vi "Close.vi"(8 "error in (no error)":errorcluster, 11 "HOTCOIL Settings":T1) -> (0 "error out":errorcluster, 3 "HOTCOIL Settings":T1)   [LabVIEW 2021, in "HotCoil.lvlib"]
uses:
  HotCoil.lvlib
  HotCoil Settings.ctl
panel:
  out "Array 2":string[](array[string])
  out "Array":string[](array[string])
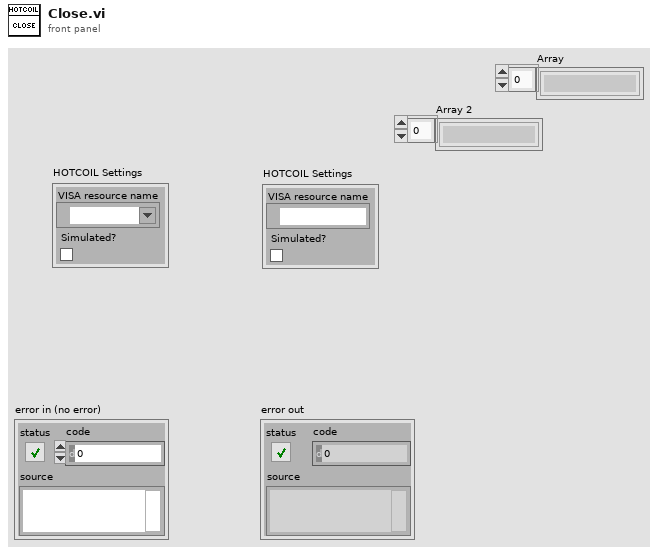
[diagram p1: front panel]
types:
  T1 = typedef "HotCoil.lvlib/HotCoil Settings.ctl" = cluster{"VISA resource name":refnum<visa-resource-name>, "Simulated?":bool}
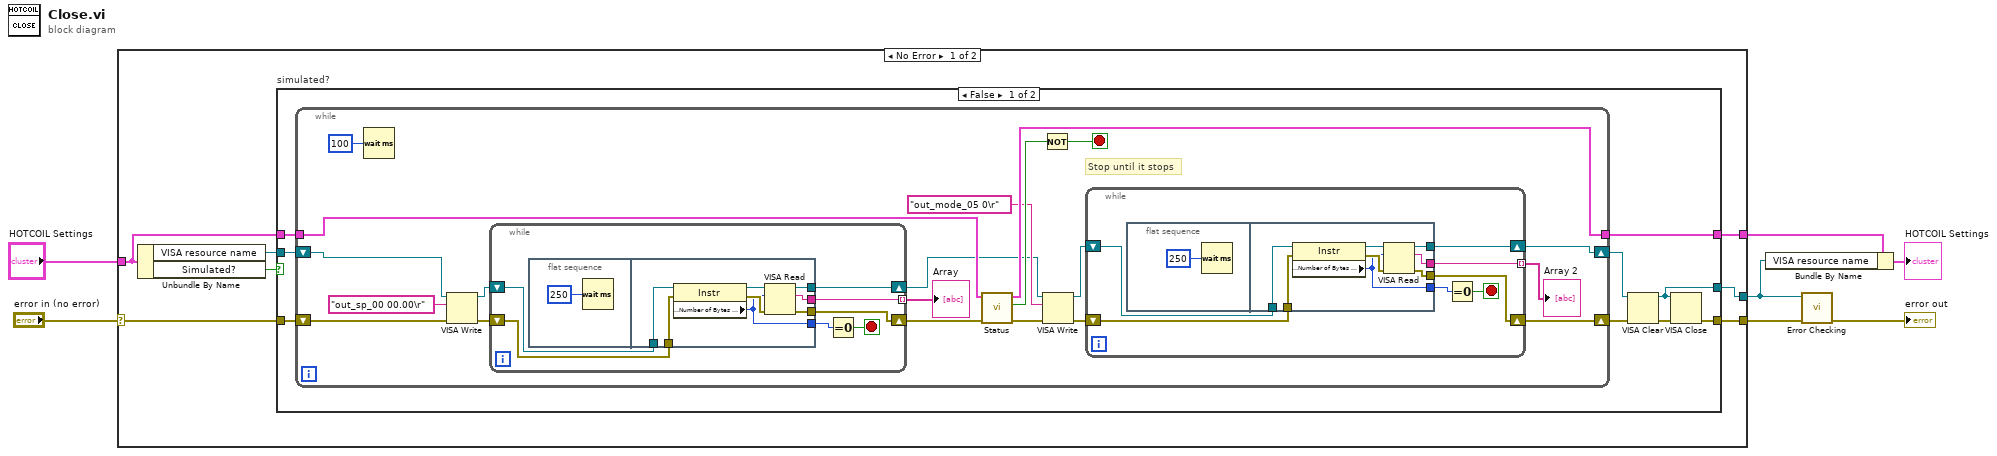
[diagram p0: block diagram]
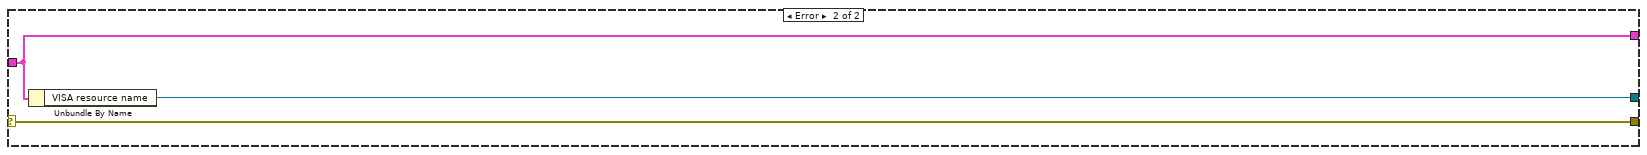
[diagram p3: hidden frame]
diagram:
  n1 = case shown="No Error" "error in (no error)" {
    selector: "error in (no error)" -> [w12 w81]
    tunnel: [w13 w81] -> w6
    tunnel: "HOTCOIL Settings" -> [w9 w79]
    tunnel: [w10 w80] -> w4
    tunnel: [w8 w79] -> w3
    frame No Error {
      n2 = Unbundle By Name(w9) -> ("VISA resource name"=w11:refnum<visa-resource-name>, "Simulated?"=w14:bool)
      n3 = case "simulated?" shown="False" w14 {
        tunnel: [w17 w78] -> w13
        tunnel: w11 -> [w22 w77]
        tunnel: w12 -> [w23 w78]
        tunnel: [w15 w77] -> w10
        tunnel: w9 -> [w21 w76]
        tunnel: [w20 w76] -> w8
        frame False {
          n4 = while {
            shift-right: [w25] -> w19
            shift-left: w23 -> [w38]
            shift-right: [w26] -> w18
            shift-left: w22 -> [w36]
            tunnel: w21 -> [w40]
            tunnel: [w41] -> w20
            stop <- w43 stop-if-true
            # "Stop until it stops"
            n5 = Wait (ms)(milliseconds to wait=u32 100) -> ()  [unwired: 1 out]
            n6 = VISA Write(VISA resource name=w36, write buffer="out_sp_00 00.00\r", error in (no error)=w38) -> (VISA resource name out=w35:refnum<visa-resource-name>, error out=w34:errorcluster)  [unwired: 1 out]
            n7 = while {
              shift-right: [w66] -> w29
              shift-left: w35 -> [w61]
              shift-right: [w65] -> w33
              shift-left: w34 -> [w60]
              tunnel: [w62] -> w32 mode=indexing
              stop <- w63 stop-if-true
              n8 = flat-sequence {
                tunnel: [w75] -> w65
                tunnel: [w74] -> w62
                tunnel: [w73] -> w66
                tunnel: [w68] -> w64
                tunnel: w61 -> [w72]
                tunnel: w60 -> [w71]
                frame #0 {
                  n9 = Wait (ms)(milliseconds to wait=u32 250) -> ()  [unwired: 1 out]
                }
                frame #1 {
                  n10 = property class="Instr"(reference=w72, error in=w71) -> (reference out=w70:refnum<visa-resource-name>, error out=w69:errorcluster, "Serial Settings:Number of Bytes at Serial Port"=w68:u32)
                  n11 = VISA Read(VISA resource name=w70, byte count=w68, error in (no error)=w69) -> (VISA resource name out=w73:refnum<visa-resource-name>, read buffer=w74:string, error out=w75:errorcluster)  [unwired: 1 out]
                }
              }
              n12 = Equal To 0?(x=w64) -> (x = 0?=w63:bool)
            }
            "Array" <- w32
            n13 = call "Status.vi"("error in (no error)"=w33, "HotCoil Settings In"=w40) -> ("error out"=w31:errorcluster, "Running"=w42:bool, "HotCoil Settings Out"=w41:T1)  [unwired: 5 in, 2 out]
            n14 = Not(x=w42) -> (.not. x?=w43:bool)
            n15 = VISA Write(VISA resource name=w29, write buffer="out_mode_05 0\r", error in (no error)=w31) -> (VISA resource name out=w28:refnum<visa-resource-name>, error out=w27:errorcluster)  [unwired: 1 out]
            n16 = while {
              shift-right: [w50] -> w26
              shift-left: w28 -> [w45]
              shift-right: [w49] -> w25
              shift-left: w27 -> [w44]
              tunnel: [w46] -> w24 mode=indexing
              stop <- w47 stop-if-true
              n17 = flat-sequence {
                tunnel: [w59] -> w49
                tunnel: [w58] -> w46
                tunnel: [w57] -> w50
                tunnel: [w52] -> w48
                tunnel: w45 -> [w56]
                tunnel: w44 -> [w55]
                frame #0 {
                  n18 = Wait (ms)(milliseconds to wait=u32 250) -> ()  [unwired: 1 out]
                }
                frame #1 {
                  n19 = property class="Instr"(reference=w56, error in=w55) -> (reference out=w54:refnum<visa-resource-name>, error out=w53:errorcluster, "Serial Settings:Number of Bytes at Serial Port"=w52:u32)
                  n20 = VISA Read(VISA resource name=w54, byte count=w52, error in (no error)=w53) -> (VISA resource name out=w57:refnum<visa-resource-name>, read buffer=w58:string, error out=w59:errorcluster)  [unwired: 1 out]
                }
              }
              n21 = Equal To 0?(x=w48) -> (x = 0?=w47:bool)
            }
            "Array 2" <- w24
          }
          n22 = VISA Clear(VISA resource name=w18, error in (no error)=w19) -> (VISA resource name out=w15:refnum<visa-resource-name>, error out=w16:errorcluster)
          n23 = VISA Close(VISA resource name=w15, error in (no error)=w16) -> (error out=w17:errorcluster)
        }
        frame True {
        }
      }
    }
    frame Error {
      n24 = Unbundle By Name(w79) -> ("VISA resource name"=w80:refnum<visa-resource-name>)
    }
  }
  n25 = Bundle By Name(cluster=w3, "VISA resource name"=w4) -> (→"HOTCOIL Settings":T1)
  n26 = call "Error Checking.vi"("error in (no error)"=w6, "VISA resource name"=w4) -> ("error out"=→"error out":errorcluster)  [unwired: 7 in, 2 out]
